vi "Query Capabilities.vi"   [LabVIEW 2012, in "NH Research Regenerative Test Series.lvlib"]
doc: "Returns various capabilities of the module."
uses:
  <instrlib>/NH Research Regenerative Test Series/NH Research Regenerative Test Series.lvlib
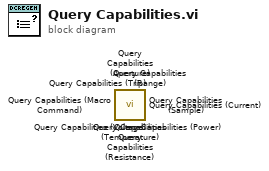
[diagram p0: block diagram]
diagram:
  n1 = call <instrlib>:"Query Capabilities (Temperature).vi"() -> ()  [unwired: 13 in, 3 out]
  n2 = call <instrlib>:"Query Capabilities (Range).vi"() -> ()  [unwired: 13 in, 3 out]
  n3 = call <instrlib>:"Query Capabilities (Macro Command).vi"() -> ()  [unwired: 11 in, 5 out]
  n4 = call <instrlib>:"Query Capabilities (Sample).vi"() -> ()  [unwired: 11 in, 5 out]
  n5 = call <instrlib>:"Query Capabilities (Trip).vi"() -> ()  [unwired: 12 in, 4 out]
  n6 = call <instrlib>:"Query Capabilities (Aperture).vi"() -> ()  [unwired: 12 in, 4 out]
  n7 = call <instrlib>:"Query Capabilities (Resistance).vi"() -> ()  [unwired: 13 in, 3 out]
  n8 = call <instrlib>:"Query Capabilities (Power).vi"() -> ()  [unwired: 13 in, 3 out]
  n9 = call <instrlib>:"Query Capabilities (Current).vi"() -> ()  [unwired: 13 in, 3 out]
  n10 = call <instrlib>:"Query Capabilities (Voltage).vi"() -> ()  [unwired: 13 in, 3 out]
